vi "rspvtd_Record Status to Caller.vi"(8 "error in":errorcluster, 11 "Data in":variant) -> (0 "error out":errorcluster, 3 "Data out":T1)   [LabVIEW 2023, in "Registration.lvclass"]
doc: "This VI converts variant data contained in the associated <b>Public API Response</b> message to its correct data type.\n---"
uses:
  Registration.lvclass
  Registration.lvclass/Registration.ctl
  rsp_Record Status to Caller.ctl
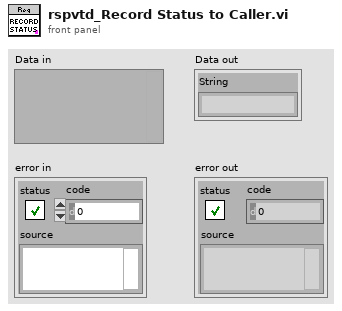
[diagram p1: front panel]
types:
  T1 = typedef "Registration.lvclass/rsp_Record Status to Caller.ctl" = cluster{"String":string}
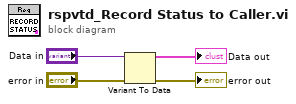
[diagram p0: block diagram]
diagram:
  n1 = Variant To Data(error in="error in", Variant="Data in") -> (data=→"Data out":T1, error out=→"error out":errorcluster)  [unwired: 1 in]
